vi "FL_Decode_RAW_to_DEC.vi"(3 "Input array of timestamps":timestamp[](array[timestamp]), 4 "Half-height of the sensor board":sgl=125.0, 5 "Half-width of the sensor board":sgl=137.5, 6 "Sensors grid step":sgl=25.0, 7 "read buffer":string) -> (0 "Output timestamp":timestamp, 1 "DEC output":sgl[](array[numeric]))   [LabVIEW 2016]
panel:
  out "offset past match":i32
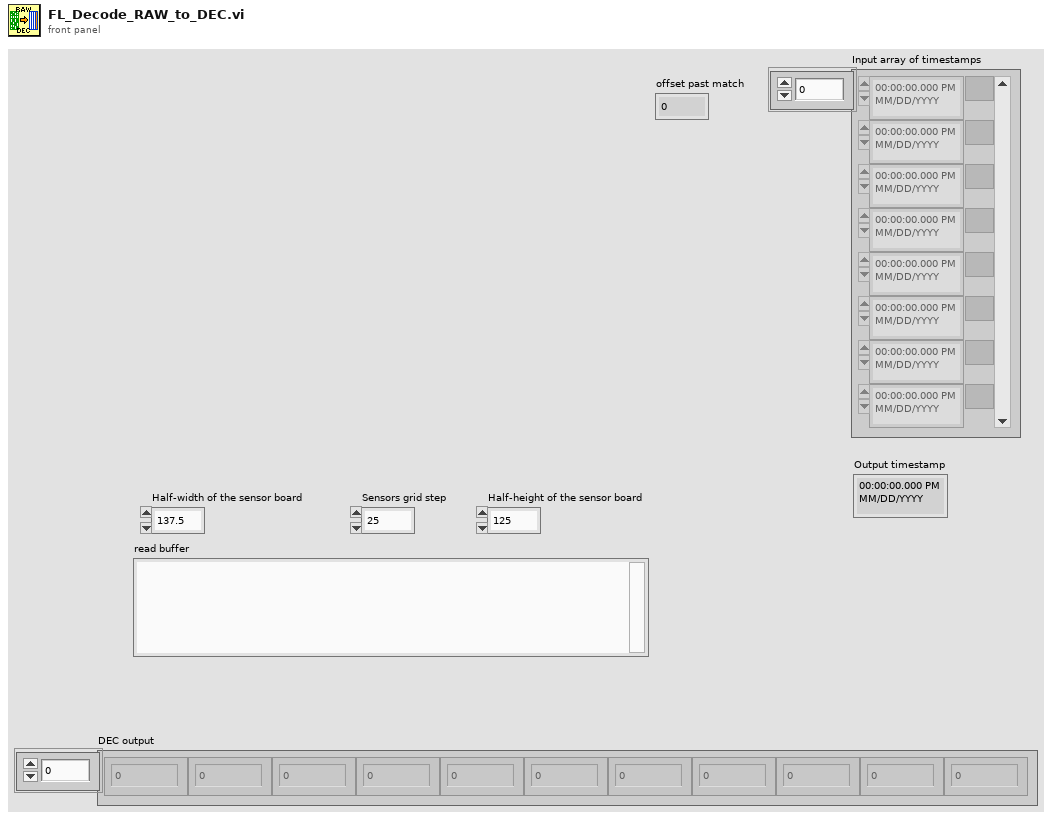
[diagram p1: front panel]
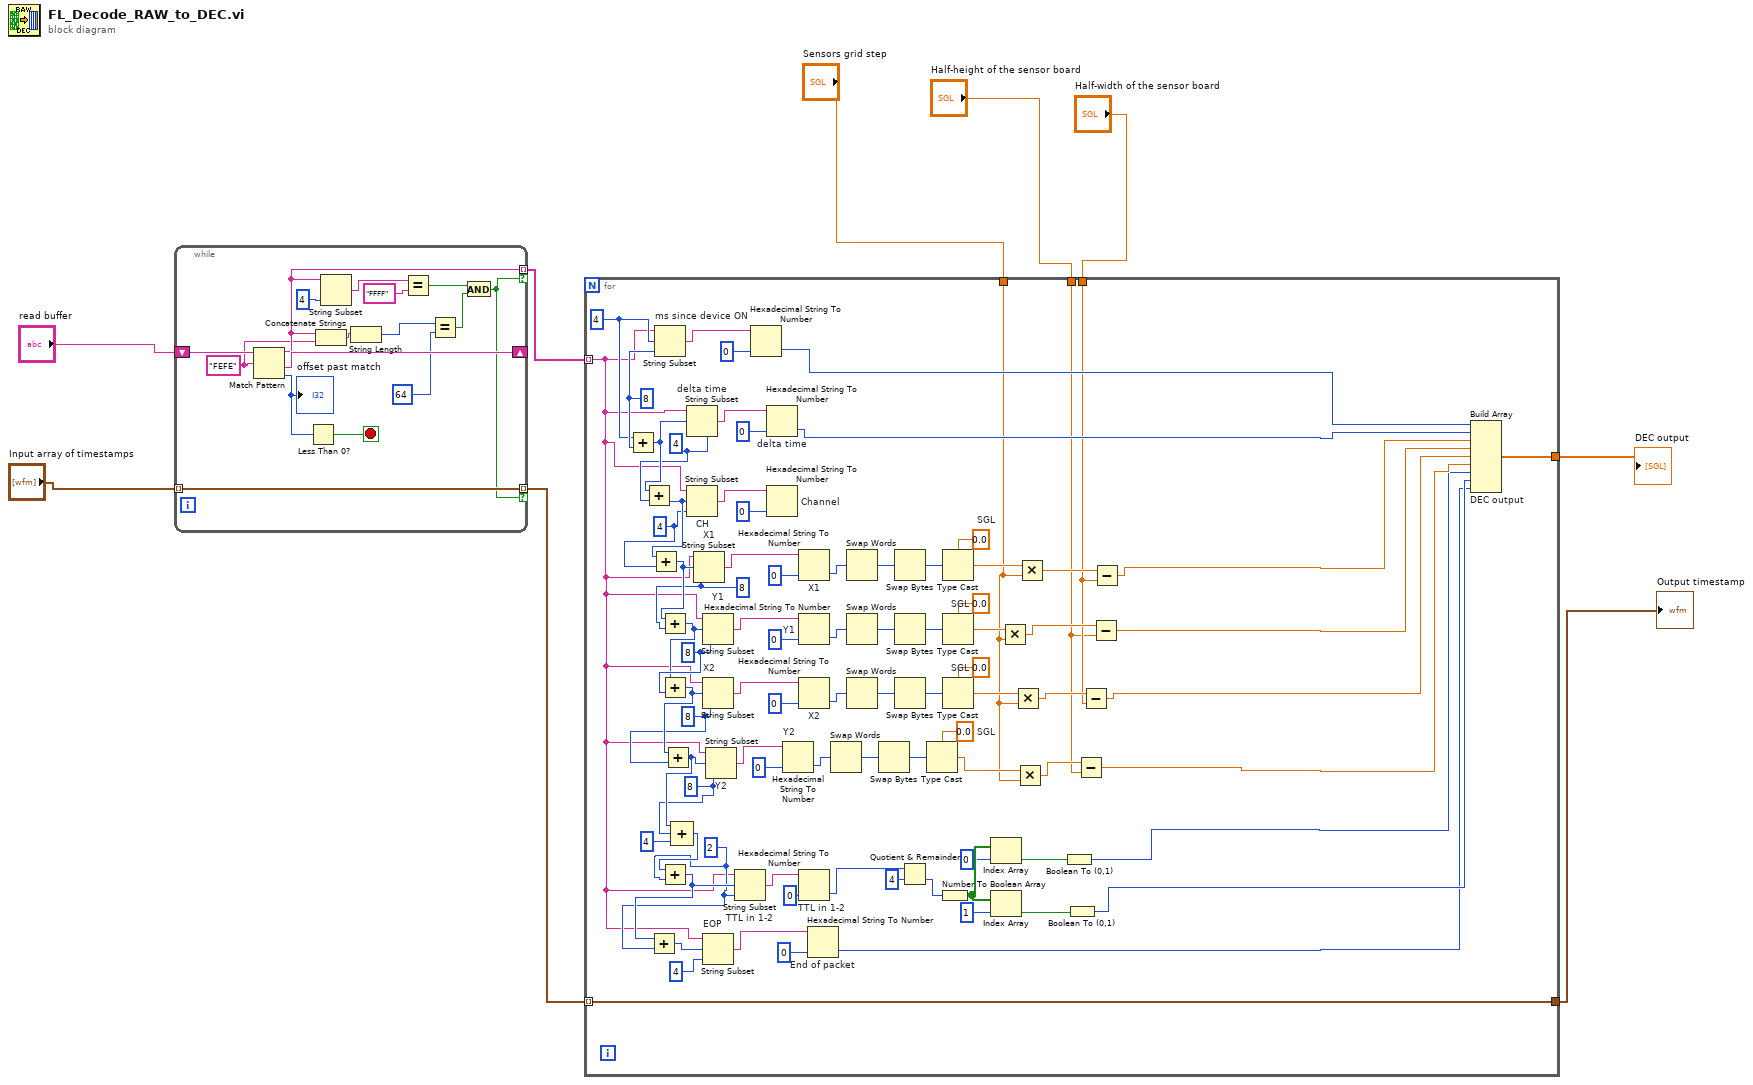
[diagram p0: block diagram]
diagram:
  n1 = while {
    shift-right: [w24] -> _
    shift-left: "read buffer" -> [w25]
    tunnel: [w14] -> w8 mode=indexing if=w10
    tunnel: [w11] -> w2 mode=indexing if=w10
    tunnel: "Input array of timestamps" -> [w11] mode=indexing
    stop <- w22 stop-if-true
    w12 = "FEFE" ("regular expression")
    n2 = Match Pattern(string=w25, regular expression=w12) -> (before substring=w14:string, after substring=w24:string, offset past match=w23:i32)  [unwired: 1 in, 1 out]
    "offset past match" <- w23
    n3 = Less Than 0?(x=w23) -> (x < 0?=w22:bool)
    n4 = Concatenate Strings(w14, w12) -> (w13:string)
    n5 = String Subset(string=w14, length (rest)=4 ("length (rest)")) -> (substring=w20:string)  [unwired: 1 in]
    n6 = String Length(string=w13) -> (length=w18:i32)
    n7 = Equal?(x=w20, y="FFFF") -> (x = y?=w16:bool)
    n8 = Equal?(x=w18, y=64) -> (x = y?=w15:bool)
    n9 = And(x=w16, y=w15) -> (x .and. y?=w10:bool)
  }
  n10 = for {
    tunnel: w8 -> [w31] mode=indexing
    tunnel: [w30] -> w7
    tunnel: "Sensors grid step" -> [w29]
    tunnel: "Half-width of the sensor board" -> [w28]
    tunnel: "Half-height of the sensor board" -> [w27]
    tunnel: w2 -> [w26] mode=indexing
    tunnel: [w26] -> w1
    w32 = 4
    w42 = 2 ("length (rest)")
    w58 = sgl 0.0  # SGL
    w65 = sgl 0.0  # SGL
    w72 = sgl 0.0  # SGL
    w78 = sgl 0.0  # SGL
    w47 = 8 ("length (rest)")
    w91 = 8 ("length (rest)")
    w94 = 8 ("length (rest)")
    w95 = 8 ("length (rest)")
    w97 = 4 ("length (rest)")
    w99 = 4 ("length (rest)")
    w101 = 8 ("length (rest)")
    n11 = Add(x=w32, y=w101) -> (x+y=w100:i32)
    n12 = Add(x=w100, y=w99) -> (x+y=w98:i32)
    n13 = Add(x=w98, y=w97) -> (x+y=w96:i32)
    n14 = String Subset "ms since device ON"(string=w31, offset (0)=w32, length (rest)=w101) -> (substring=w88:string)
    n15 = Add(x=w96, y=w95) -> (x+y=w93:i32)
    n16 = Add(x=w93, y=w94) -> (x+y=w92:i32)
    n17 = Add(x=w92, y=w91) -> (x+y=w48:i32)
    n18 = Compound Arithmetic op=unknown(w48, w47, 4 ("value")) -> (w44:i32)
    n19 = Add(x=w44, y=w42) -> (x+y=w43:i32)
    n20 = Add(x=w43, y=w42) -> (x+y=w90:i32)
    n21 = String Subset "delta time"(string=w31, offset (0)=w100, length (rest)=w99) -> (substring=w85:string)
    n22 = String Subset "CH"(string=w31, offset (0)=w98, length (rest)=w97) -> (substring=w83:string)
    n23 = String Subset "X1"(string=w31, offset (0)=w96, length (rest)=w95) -> (substring=w82:string)
    n24 = String Subset "Y1"(string=w31, offset (0)=w93, length (rest)=w94) -> (substring=w70:string)
    n25 = String Subset "X2"(string=w31, offset (0)=w92, length (rest)=w91) -> (substring=w63:string)
    n26 = String Subset "EOP"(string=w31, offset (0)=w90, length (rest)=4 ("length (rest)")) -> (substring=w53:string)
    n27 = String Subset "Y2"(string=w31, offset (0)=w48, length (rest)=w47) -> (substring=w56:string)
    n28 = String Subset "TTL in 1-2"(string=w31, offset (0)=w43, length (rest)=w42) -> (substring=w46:string)
    n29 = Hexadecimal String To Number ("ms since ON")(string=w88, default (0uL)=u32 0 ("default (0 U32)")) -> (number=w110:u32)  [unwired: 1 in, 1 out]
    n30 = Hexadecimal String To Number "delta time"(string=w85, default (0uL)=u32 0 ("default (0 U32)")) -> (number=w109:u32)  [unwired: 1 in, 1 out]
    n31 = Hexadecimal String To Number "Channel"(string=w83, default (0uL)=u32 0 ("default (0 U32)")) -> ()  [unwired: 1 in, 2 out]
    n32 = Hexadecimal String To Number "Y2"(string=w56, default (0uL)=u32 0 ("default (0 U32)")) -> (number=w60:u32)  [unwired: 1 in, 1 out]
    n33 = Hexadecimal String To Number "X1"(string=w82, default (0uL)=u32 0 ("default (0 U32)")) -> (number=w80:u32)  [unwired: 1 in, 1 out]
    n34 = Hexadecimal String To Number "Y1"(string=w70, default (0uL)=u32 0 ("default (0 U32)")) -> (number=w74:u32)  [unwired: 1 in, 1 out]
    n35 = Hexadecimal String To Number "X2"(string=w63, default (0uL)=u32 0 ("default (0 U32)")) -> (number=w67:u32)  [unwired: 1 in, 1 out]
    n36 = Hexadecimal String To Number "TTL in 1-2"(string=w46, default (0uL)=u32 0 ("default (0 U32)")) -> (number=w39:u32)  [unwired: 1 in, 1 out]
    n37 = Hexadecimal String To Number "End of packet"(string=w53, default (0uL)=u32 0 ("default (0 U32)")) -> (number=w102:u32)  [unwired: 1 in, 1 out]
    n38 = Swap Words(1:w60) -> (0:w59:u32)
    n39 = Swap Words(1:w80) -> (0:w79:u32)
    n40 = Swap Words(1:w74) -> (0:w73:u32)
    n41 = Swap Words(1:w67) -> (0:w66:u32)
    n42 = Swap Bytes(anything=w59) -> (byte swapped=w57:u32)
    n43 = Swap Bytes(anything=w79) -> (byte swapped=w77:u32)
    n44 = Swap Bytes(anything=w73) -> (byte swapped=w71:u32)
    n45 = Swap Bytes(anything=w66) -> (byte swapped=w64:u32)
    n46 = Quotient & Remainder(x=w39, y=u32 4) -> (floor(x/y)=w38:u32)  [unwired: 1 out]
    n47 = Type Cast(type=w58, x=w57) -> (*(type *) &x=w55:sgl)
    n48 = Number To Boolean Array(number=w38) -> (Boolean array=w37:bool[])
    n49 = Type Cast(type=w78, x=w77) -> (*(type *) &x=w76:sgl)
    n50 = Type Cast(type=w72, x=w71) -> (*(type *) &x=w69:sgl)
    n51 = Type Cast(type=w65, x=w64) -> (*(type *) &x=w62:sgl)
    n52 = Index Array(array=w37, index=0) -> (element=w34:bool)
    n53 = Index Array(array=w37, index=1) -> (element=w33:bool)
    n54 = Multiply(x=w69, y=w29) -> (x*y=w50:sgl)
    n55 = Multiply(x=w62, y=w29) -> (x*y=w51:sgl)
    n56 = Multiply(x=w55, y=w29) -> (x*y=w49:sgl)
    n57 = Multiply(x=w76, y=w29) -> (x*y=w52:sgl)
    n58 = Boolean To (0,1)(Boolean=w34) -> (0, 1=w104:i16)
    n59 = Boolean To (0,1)(Boolean=w33) -> (0, 1=w103:i16)
    n60 = Subtract(x=w49, y=w27) -> (x-y=w105:sgl)
    n61 = Subtract(x=w51, y=w28) -> (x-y=w106:sgl)
    n62 = Subtract(x=w50, y=w27) -> (x-y=w107:sgl)
    n63 = Subtract(x=w52, y=w28) -> (x-y=w108:sgl)
    n64 = Build Array "DEC output"(w110, w109, w108, w107, w106, w105, w104, w103, w102) -> (w30:sgl[])
  }
  "DEC output" <- w7
  "Output timestamp" <- w1
